vi "AccelnetTorqueInScale.vi"(1 "Torque (Raw from drive)":i16) -> (0 "Torque (Nm)":dbl)   [LabVIEW 2018]
uses:
  Clusters/SimulationConstants.ctl
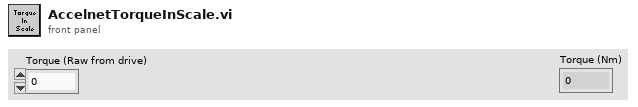
[diagram p1: front panel]
types:
  T1 = typedef "SimulationConstants.ctl" = cluster{"nGear":dbl, "rotorRadius":sgl, "numBlades":i32, "scaleFactor":dbl, "roscoInitMinSpeed_rad_s":dbl, "roscoInitMinTorqueFS_Nm":dbl, "beckhoff16bit":dbl, "beckhoff24BitExt":i32, "BX824Bit":i32, "rotorTorqueScale_Nm_V":dbl, "rotorTorqueOfst_Nm":dbl, "rangeEL3104V":dbl, "nacelleAccELM3604V":dbl, "nacelleAccScaleX_m_s2_V":dbl, "nacelleAccOfstX_m_s2":dbl, "nacelleAccScaleY_m_s2_V":dbl, "nacelleAccOfstY_m_s2":dbl, "nacelleAccScaleZ_m_s2_V":dbl, "nacelleAccOfstZ_m_s2":dbl, "cyberGearRatio":dbl, "cyberLinesPerRev":dbl, "cyberRatedTorque":dbl, "towerTopForceScale":dbl, "towerTopTorqueScale":dbl, "plcSetpointScaling_norm2VFD":dbl, "towerBotScaleMy_Nm_V":dbl, "towerBotOfstMy_Nm":dbl, "towerTopScaleXaxis_N_V":dbl, "towerTopOfstXaxis_N":dbl, "towerTopScaleYaxis_N_V":dbl, "towerTopOfstYaxis_N":dbl, "pitchFlagOffset_deg":dbl, "anemWindSpeedScaleU_m_s_m_s":dbl, "anemWindSpeedOfstU_m_s":dbl, "anemWindSpeedScaleV_m_s_m_s":dbl, "anemWindSpeedOfstV_m_s":dbl, "anemWindSpeedScaleW_m_s_m_s":dbl, "anemWindSpeedOfstW_m_s":dbl, "anemWindSpeedScaleTSI1_m_s_V":dbl, "anemWindSpeedOfstTSI1_m_s":dbl, "anemWindSpeedScaleTSI3_m_s_V":dbl, "anemWindSpeedOfstTSI3_m_s":dbl, "anemWindSpeedScaleXProbeA1C0":dbl, "anemWindSpeedScaleXProbeA1C1":dbl, "anemWindSpeedScaleXProbeA1C2":dbl, "anemWindSpeedScaleXProbeA1C3":dbl, "anemWindSpeedScaleXProbeA1C4":dbl, "anemWindSpeedOfstXProbeA1_m_s":dbl, "anemWindSpeedScaleXProbeA2C0":dbl, "anemWindSpeedScaleXProbeA2C1":dbl, "anemWindSpeedScaleXProbeA2C2":dbl, "anemWindSpeedScaleXProbeA2C3":dbl, "anemWindSpeedScaleXProbeA2C4":dbl, "anemWindSpeedOfstXProbeA2_m_s":dbl, "anemWindSpeedScaleXProbeC1C0":dbl, "anemWindSpeedScaleXProbeC1C1":dbl, "anemWindSpeedScaleXProbeC1C2":dbl, "anemWindSpeedScaleXProbeC1C3":dbl, "anemWindSpeedScaleXProbeC1C4":dbl, "anemWindSpeedOfstXProbeC1_m_s":dbl, "anemWindSpeedScaleXProbeC2C0":dbl, "anemWindSpeedScaleXProbeC2C1":dbl, "anemWindSpeedScaleXProbeC2C2":dbl, "anemWindSpeedScaleXProbeC2C3":dbl, "anemWindSpeedScaleXProbeC2C4":dbl, "anemWindSpeedOfstXProbeC2_m_s":dbl, "anemWindSpeedScaleXProbeD1C0":dbl, "anemWindSpeedScaleXProbeD1C1":dbl, "anemWindSpeedScaleXProbeD1C2":dbl, "anemWindSpeedScaleXProbeD1C3":dbl, "anemWindSpeedScaleXProbeD1C4":dbl, "anemWindSpeedOfstXProbeD1_m_s":dbl, "anemWindSpeedScaleXProbeD2C0":dbl, "anemWindSpeedScaleXProbeD2C1":dbl, "anemWindSpeedScaleXProbeD2C2":dbl, "anemWindSpeedScaleXProbeD2C3":dbl, "anemWindSpeedScaleXProbeD2C4":dbl, "anemWindSpeedOfstXProbeD2_m_s":dbl, "anemWindSpeedOfstHw3_m_s":dbl, "anemWindSpeedScaleHw3_m_s_V":dbl, "probeAOfstX_mm":dbl, "probeAOfstY_mm":dbl, "probeAOfstZ_mm":dbl, "probeTSIOfstX_mm":dbl, "probeTSIOfstY_mm":dbl, "probeTSIOfstZ_mm":dbl, "probeBOfstX_mm":dbl, "probeBOfstY_mm":dbl, "probeBOfstZ_mm":dbl}
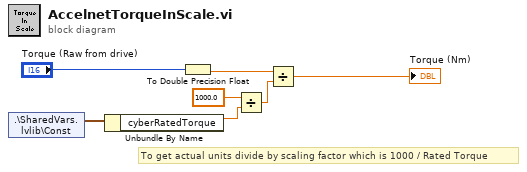
[diagram p0: block diagram]
diagram:
  # "To get actual units divide by scaling factor which is 1000 / Rated Torque"
  n1 = shared-variable ".\\SharedVars.lvlib\\Const"() -> (w4:T1)  [unwired: 1 in, 1 out]
  n2 = Unbundle By Name(w4) -> ("cyberRatedTorque"=w2:dbl)
  n3 = To Double Precision Float(number="Torque (Raw from drive)") -> (double precision float=w6:dbl)
  n4 = Divide(x=1000.0, y=w2) -> (x/y=w1:dbl)
  n5 = Divide(x=w6, y=w1) -> (x/y=→"Torque (Nm)":dbl)
